vi "initialize Session Data.vi"(0 "OBJ - Session in":refnum<class "Config Data.lvclass">, 11 "error in":errorcluster) -> (4 "OBJ - Session out":refnum<class "Config Data.lvclass">, 15 "error out":errorcluster)   [LabVIEW 2015, in "Config Data.lvclass"]
doc: "OVERRIDE VI\nPlaceholder for decendant sessions to initialize and set their default values"
uses:
  Config Data.lvclass
  Config Data.lvclass/Config Data.ctl
  <vilib>/Utility/config.llb/NI_LVConfig.lvlib
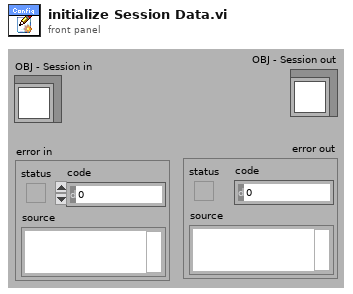
[diagram p1: front panel]
types:
  T1 = typedef "NI_LVConfig.lvlib/Config Data RefNum.ctl" = refnum<k1>
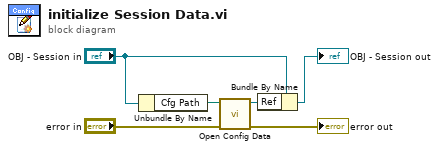
[diagram p0: block diagram]
diagram:
  n1 = Unbundle By Name("OBJ - Session in") -> ("Cfg Path"=w6:path)
  n2 = call <vilib>:"Open Config Data.vi"("error in (no error)"="error in", "configuration file path"=w6) -> ("error out"=→"error out":errorcluster, "refnum"=w4:T1)  [unwired: 7 in, 1 out]
  n3 = Bundle By Name(cluster="OBJ - Session in", "Ref"=w4) -> (→"OBJ - Session out":refnum<class "Config Data.lvclass">)
